vi "VoltToPixel.vi"(8 "1/(QPDY/px)":sgl, 9 "Normalized Y":sgl, 10 "1/(QPDX/px)":sgl, 11 "Normalized X":sgl) -> (0 "Ypx":sgl, 3 "Xpx":sgl)   [LabVIEW 2019]
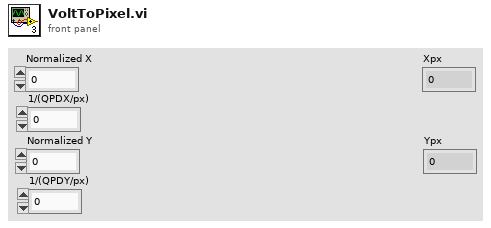
[diagram p1: front panel]
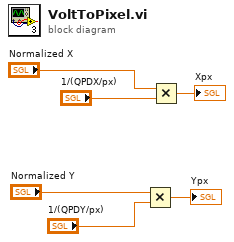
[diagram p0: block diagram]
diagram:
  n1 = Multiply(x="Normalized Y", y="1/(QPDY/px)") -> (x*y=→"Ypx":sgl)
  n2 = Multiply(x="Normalized X", y="1/(QPDX/px)") -> (x*y=→"Xpx":sgl)
